vi "Header String (I64).vi"(10 "Value":i64, 11 "Name":string) -> (3 "Header":string)   [LabVIEW 2020, in "HTTP Utils.lvlib"]
uses:
  HTTP Utils.lvlib
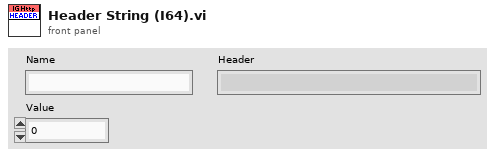
[diagram p1: front panel]
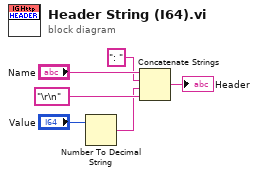
[diagram p0: block diagram]
diagram:
  n1 = Number To Decimal String(number="Value") -> (decimal integer string=w1:string)  [unwired: 1 in]
  n2 = Concatenate Strings("Name", ": " ("string"), w1, "\r\n" ("string")) -> (→"Header":string)
